vi "Teste_comunicação_mario.vi"() -> ()   [LabVIEW 2017]
panel:
  out "Estado_esteira":bool
  in  "Stop Button":bool
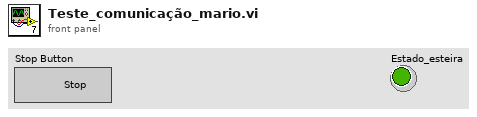
[diagram p1: front panel]
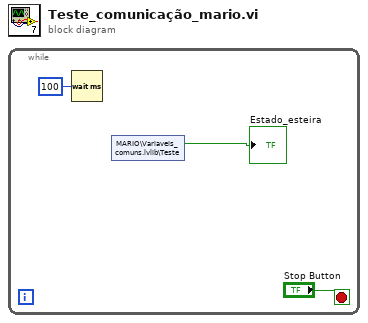
[diagram p0: block diagram]
diagram:
  n1 = while {
    stop <- "Stop Button" stop-if-true
    n2 = Wait (ms)(milliseconds to wait=u32 100) -> ()  [unwired: 1 out]
    n3 = shared-variable "MARIO\\Variaveis_comuns.lvlib\\Teste"() -> (→"Estado_esteira":bool)  [unwired: 1 in, 1 out]
  }
